vi "Make Long Class Name.vi"(10 "Short Class Name":string, 11 "Data Types Dict":variant) -> (2 "Long Class Name":string, 3 "Found":bool)   [LabVIEW 2017, in "Tree API.lvlib" / "Tree.lvclass"]
uses:
  Tree.lvclass
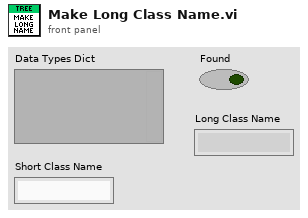
[diagram p1: front panel]
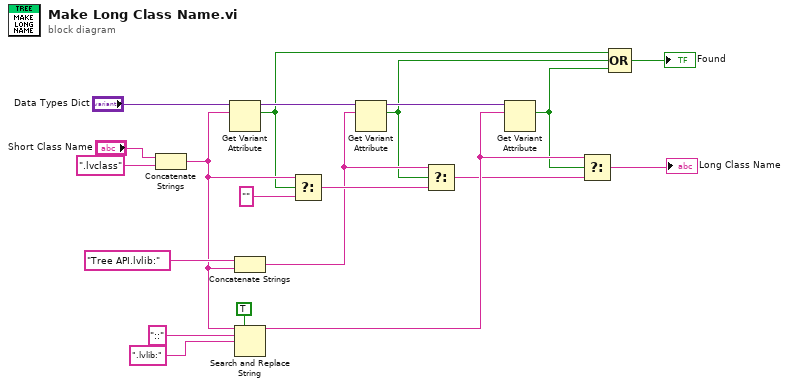
[diagram p0: block diagram]
diagram:
  n1 = Concatenate Strings("Short Class Name", ".lvclass" ("string")) -> (w13:string)
  n2 = Get Variant Attribute(Variant="Data Types Dict", name=w13) -> (duplicate Variant=w12:variant, found=w3:bool)  [unwired: 2 in, 2 out]
  n3 = Concatenate Strings("Tree API.lvlib:" ("string"), w13) -> (w8:string)
  n4 = Search and Replace String(replace all?=TRUE ("replace all? (F)"), input string=w13, search string="::" ("replace string (\"\")"), replace string=".lvlib:" ("regular expression")) -> (result string=w7:string)  [unwired: 4 in, 3 out]
  n5 = Select(t=w13, s=w3, f="") -> (s? t:f=w10:string)
  n6 = Get Variant Attribute(Variant=w12, name=w8) -> (duplicate Variant=w9:variant, found=w4:bool)  [unwired: 2 in, 2 out]
  n7 = Select(t=w8, s=w4, f=w10) -> (s? t:f=w6:string)
  n8 = Get Variant Attribute(Variant=w9, name=w7) -> (found=w5:bool)  [unwired: 2 in, 3 out]
  n9 = Select(t=w7, s=w5, f=w6) -> (s? t:f=→"Long Class Name":string)
  n10 = Compound Arithmetic op=OR(w3, w4, w5) -> (→"Found":bool)
